vi "AE - Bluetooth IRData.vi"(8 "error in (no error)":errorcluster, 11 "Wiimote":i32) -> (0 "error out":errorcluster, 3 "IRState":T1 {"Mode" items=["Off"=0, "Basic"=1, "Extended"=3, "Full"=5]})   [LabVIEW 2010]
uses:
  AE Cores/Custom Controls/WiimoteState(IR).ctl
  AE Cores/AE - Bluetooth Enum.ctl
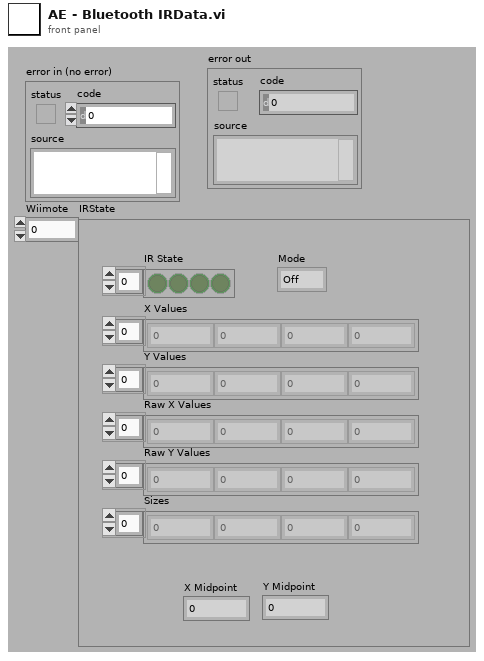
[diagram p1: front panel]
types:
  T1 = typedef "WiimoteState(IR).ctl" = cluster{"Mode":u8, "IR State":bool[], "X Values":sgl[], "Y Values":sgl[], "Raw X Values":i32[], "Raw Y Values":i32[], "Sizes":i32[], "X Midpoint":sgl, "Y Midpoint":sgl}
  T2 = typedef "AE - Bluetooth Enum.ctl" = enum16{"Initialise", "Pair All Wiimotes", "Connect All Wiimotes", "Set Rumble", "Set LED", "Get Button + Acc Data", "Get IR Data", "Get Battery", "Get Wiimote Reference", "Reorder Wiimotes", "devReport"}
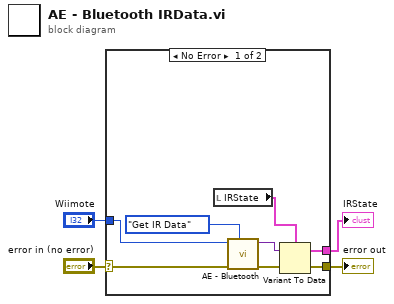
[diagram p0: block diagram]
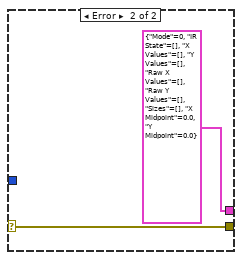
[diagram p2: hidden frame]
diagram:
  n1 = case shown="No Error" "error in (no error)" {
    selector: "error in (no error)" -> [w11 w14]
    tunnel: [w8 w14] -> w3
    tunnel: "Wiimote" -> [w10 _]
    tunnel: [w5 T1 {"Mode"=0, "IR State"=[], "X Values"=[], "Y Values"=[], "Raw X Values"=[], "Raw Y Values"=[], "Sizes"=[], "X Midpoint"=0.0, "Y Midpoint"=0.0} ("IRState")] -> w1
    frame No Error {
      n2 = local read "IRState"() -> (w6:T1)
      n3 = call "AE - Bluetooth.vi"("Enum"=AE_-_Bluetooth_Enum."Get IR Data", "error in (no error)"=w11, "Variant In"=w10) -> ("error out"=w9:errorcluster, "Variant Out"=w7:variant)  [unwired: 6 in, 1 out]
      n4 = Variant To Data(error in=w9, Variant=w7, type=w6) -> (error out=w8:errorcluster, data=w5:T1)
    }
    frame Error {
    }
  }
  "error out" <- w3
  "IRState" <- w1
